vi "NTJ_TCP_WriteWithRetries.vi"(9 "Msg Buffer":string, 11 "TCP Network Connection in":refnum<k5>) -> (0 "error out":errorcluster, 3 "bytes written":i32)   [LabVIEW 2019]
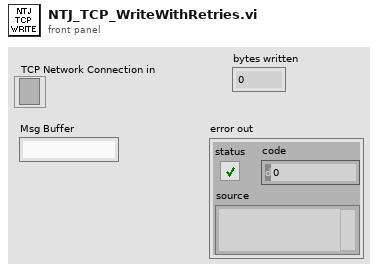
[diagram p1: front panel]
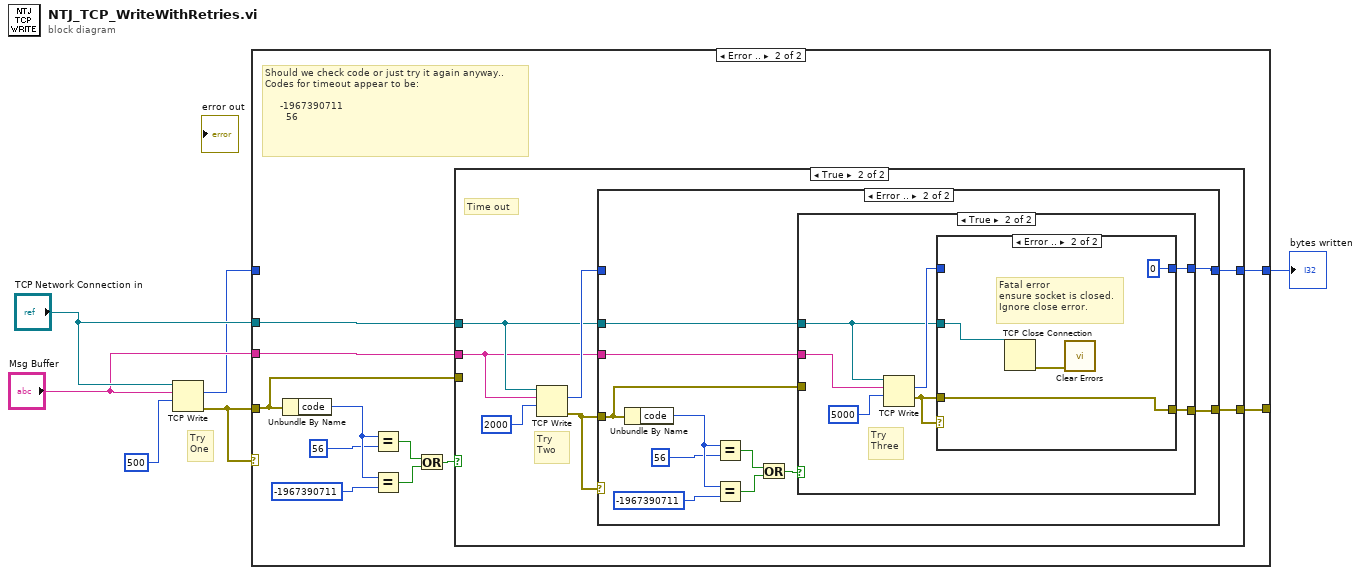
[diagram p0: block diagram]
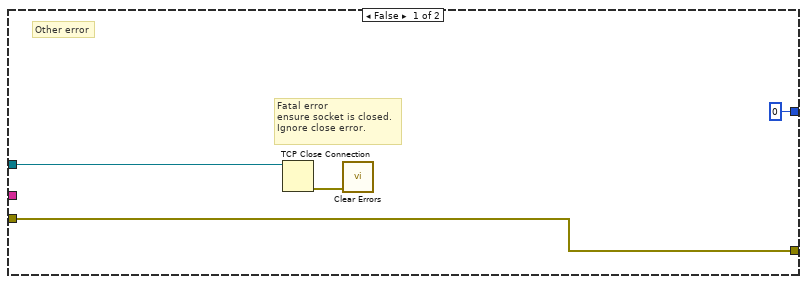
[diagram p3: hidden frame]
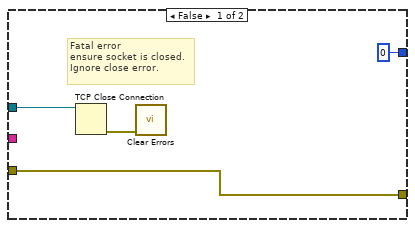
[diagram p5: hidden frame]
diagram:
  # "Try\nOne"
  n1 = TCP Write(connection ID="TCP Network Connection in", data in="Msg Buffer", 9:500 ("timeout ms (25000)")) -> (bytes written=w2:i32, error out=w5:errorcluster)  [unwired: 1 in, 1 out]
  n2 = case shown="Error .." w5 {
    tunnel: w5 -> [w8 w11]
    tunnel: "TCP Network Connection in" -> [_ w13]
    tunnel: "Msg Buffer" -> [_ w12]
    tunnel: w2 -> [w7 _]
    tunnel: [w8 w10] -> _
    tunnel: [w7 w9] -> w1
    frame No Error {
    }
    frame Error {
      # "Should we check code or just try it again anyway..\nCodes for timeout appear to be:\n\n     -1967390711\n       56"
      n3 = Unbundle By Name(w11) -> ("code"=w19:i32)
      n4 = Equal?(x=w19, y=56) -> (x = y?=w16:bool)
      n5 = Equal?(x=w19, y=-1967390711) -> (x = y?=w15:bool)
      n6 = Or(x=w16, y=w15) -> (x .or. y?=w14:bool)
      n7 = case shown="True" w14 {
        tunnel: w13 -> [w22 w25]
        tunnel: w12 -> [_ w24]
        tunnel: w11 -> [w23 _]
        tunnel: [w23 w26] -> w10
        tunnel: [0 ("bytes written") w27] -> w9
        frame False {
          # "Fatal error\nensure socket is closed.\nIgnore close error."
          # "Other error"
          n8 = TCP Close Connection(connection ID=w22) -> (error out=w21:errorcluster)  [unwired: 2 in, 1 out]
          n9 = call <vilib>:"Clear Errors.vi"("error in (no error)"=w21) -> ()  [unwired: 5 in, 2 out]
        }
        frame True {
          # "Try\nTwo"
          # "Time out"
          n10 = TCP Write(connection ID=w25, data in=w24, 9:2000 ("timeout ms (25000)")) -> (bytes written=w28:i32, error out=w29:errorcluster)  [unwired: 1 in, 1 out]
          n11 = case shown="Error .." w29 {
            tunnel: w29 -> [w31 w35]
            tunnel: [w32 w33] -> w27
            tunnel: w28 -> [w32 _]
            tunnel: [w31 w36] -> w26
            tunnel: w25 -> [_ w37]
            tunnel: w24 -> [_ w34]
            frame No Error {
            }
            frame Error {
              n12 = Unbundle By Name(w35) -> ("code"=w43:i32)
              n13 = Equal?(x=w43, y=56) -> (x = y?=w40:bool)
              n14 = Equal?(x=w43, y=-1967390711) -> (x = y?=w39:bool)
              n15 = Or(x=w40, y=w39) -> (x .or. y?=w38:bool)
              n16 = case shown="True" w38 {
                tunnel: w37 -> [w46 w48]
                tunnel: [w45 w52] -> w36
                tunnel: w35 -> [w45 _]
                tunnel: w34 -> [_ w53]
                tunnel: [0 ("bytes written") w49] -> w33
                frame False {
                  # "Fatal error\nensure socket is closed.\nIgnore close error."
                  n17 = TCP Close Connection(connection ID=w46) -> (error out=w47:errorcluster)  [unwired: 2 in, 1 out]
                  n18 = call <vilib>:"Clear Errors.vi"("error in (no error)"=w47) -> ()  [unwired: 5 in, 2 out]
                }
                frame True {
                  # "Try\nThree"
                  n19 = TCP Write(connection ID=w48, data in=w53, 9:5000 ("timeout ms (25000)")) -> (bytes written=w50:i32, error out=w51:errorcluster)  [unwired: 1 in, 1 out]
                  n20 = case shown="Error .." w51 {
                    tunnel: [w56 w60] -> w52
                    tunnel: w51 -> [w56 w60]
                    tunnel: [w55 0 ("bytes written")] -> w49
                    tunnel: w50 -> [w55 _]
                    tunnel: w48 -> [_ w58]
                    frame No Error {
                    }
                    frame Error {
                      # "Fatal error\nensure socket is closed.\nIgnore close error."
                      n21 = TCP Close Connection(connection ID=w58) -> (error out=w59:errorcluster)  [unwired: 2 in, 1 out]
                      n22 = call <vilib>:"Clear Errors.vi"("error in (no error)"=w59) -> ()  [unwired: 5 in, 2 out]
                    }
                  }
                }
              }
            }
          }
        }
      }
    }
  }
  "bytes written" <- w1
